vi "MeasureBreakdown.vi"(1 "Microsites":refnum<k24>, 2 "Junction Name":string, 7 ".NET Refnum":refnum<k24>, 9 "Function":string, 12 "appended path":path, 13 "new file path (Not A Path if cancelled)":path, 14 "UiDefinition":T1) -> (15 "error out":errorcluster)   [LabVIEW 2020]
uses:
  UIReferences.ctl
  D:/LabviewDXFViewer/LabviewDXFViewer/bin/Release/LabviewDXFViewer.exe
  LabviewDXFViewer/bin/Release/LabviewDXFViewer.exe
  <vilib>/Utility/file.llb/Write Delimited Spreadsheet (DBL).vi
  <vilib>/Utility/file.llb/Write Delimited Spreadsheet (string).vi
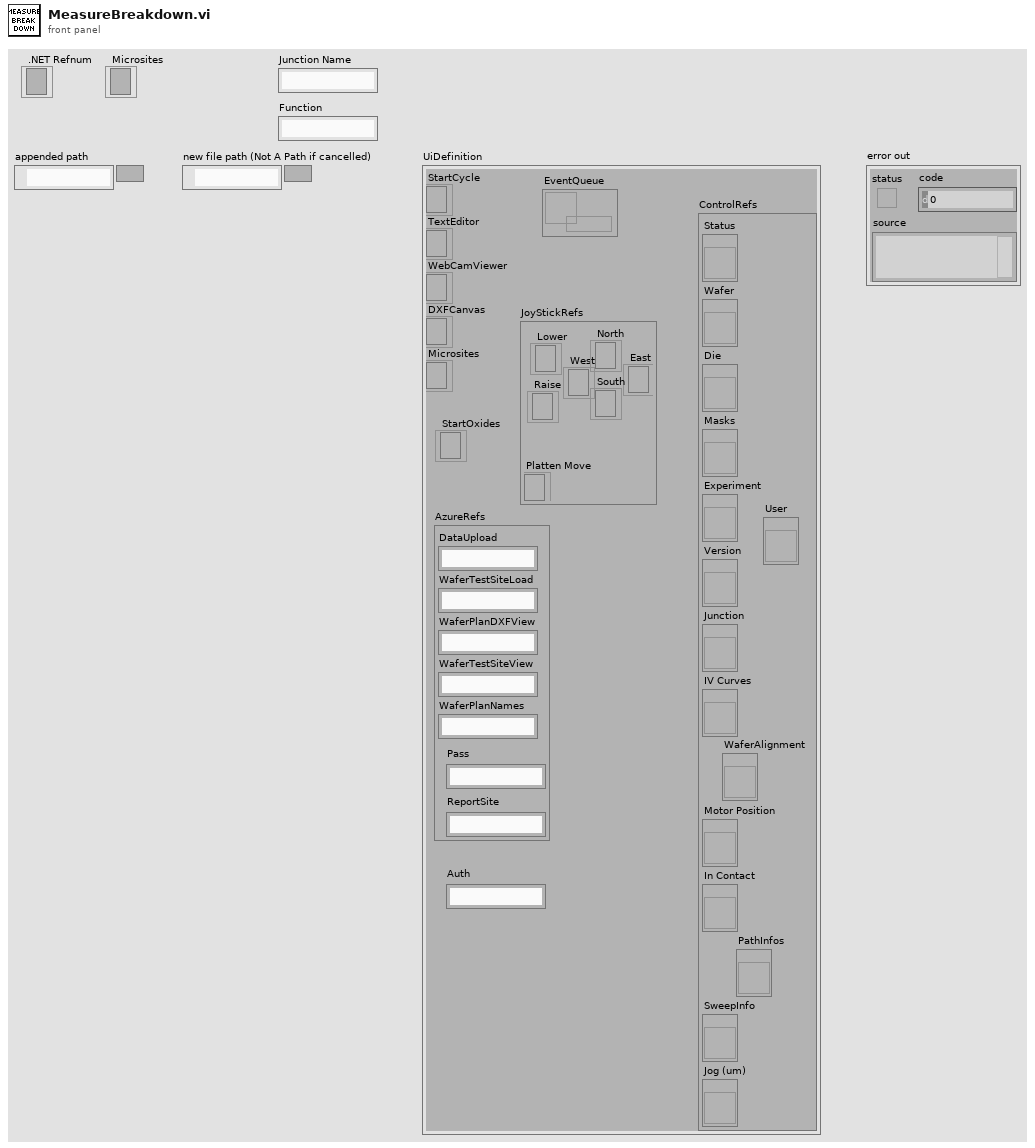
[diagram p1: front panel]
types:
  T1 = typedef "UIReferences.ctl" = cluster{"StartCycle":refnum<k24>, "TextEditor":refnum<k24>, "WebCamViewer":refnum<k24>, "DXFCanvas":refnum<k24>, "Microsites":refnum<k24>, "JoyStickRefs":cluster{"North":refnum<k24>, "Lower":refnum<k24>, "Raise":refnum<k24>, "Platten Move":refnum<k24>, "West":refnum<k24>, "East":refnum<k24>, "South":refnum<k24>}, "AzureRefs":cluster{"DataUpload":string, "WaferTestSiteLoad":string, "WaferPlanDXFView":string, "WaferTestSiteView":string, "WaferPlanNames":string, "Pass":string, "ReportSite":string}, "ControlRefs":cluster{"Status":refnum<vi>, "Wafer":refnum<vi>, "Die":refnum<vi>, "Masks":refnum<vi>, "Experiment":refnum<vi>, "Version":refnum<vi>, "Junction":refnum<vi>, "IV Curves":refnum<vi>, "Motor Position":refnum<vi>, "In Contact":refnum<vi>, "SweepInfo":refnum<vi>, "Jog (um)":refnum<vi>, "PathInfos":refnum<vi>, "User":refnum<vi>, "WaferAlignment":refnum<vi>}, "EventQueue":refnum<queue>, "StartOxides":refnum<k24>, "Auth":string}
  T2 = typedef "CapacitanceInfos.ctl" = cluster{"Conductance":dbl, "CapacitanceIV":dbl, "Intercept":dbl, "CapacitanceSW":dbl, "Sum":dbl, "CapacitanceInfos":T3[], "CapacitancePhase":dbl, "dC/dV":dbl, "Function":string, "OtherInfo":dbl[][]}
  T3 = typedef "CapacitanceRecord.ctl" = cluster{"Freq":dbl, "Vpp":dbl, "PhaseS":dbl, "Irms":dbl, "PhaseC":dbl, "Theta":dbl, "VDrive":dbl, "Capacitance":dbl, "Other":dbl}
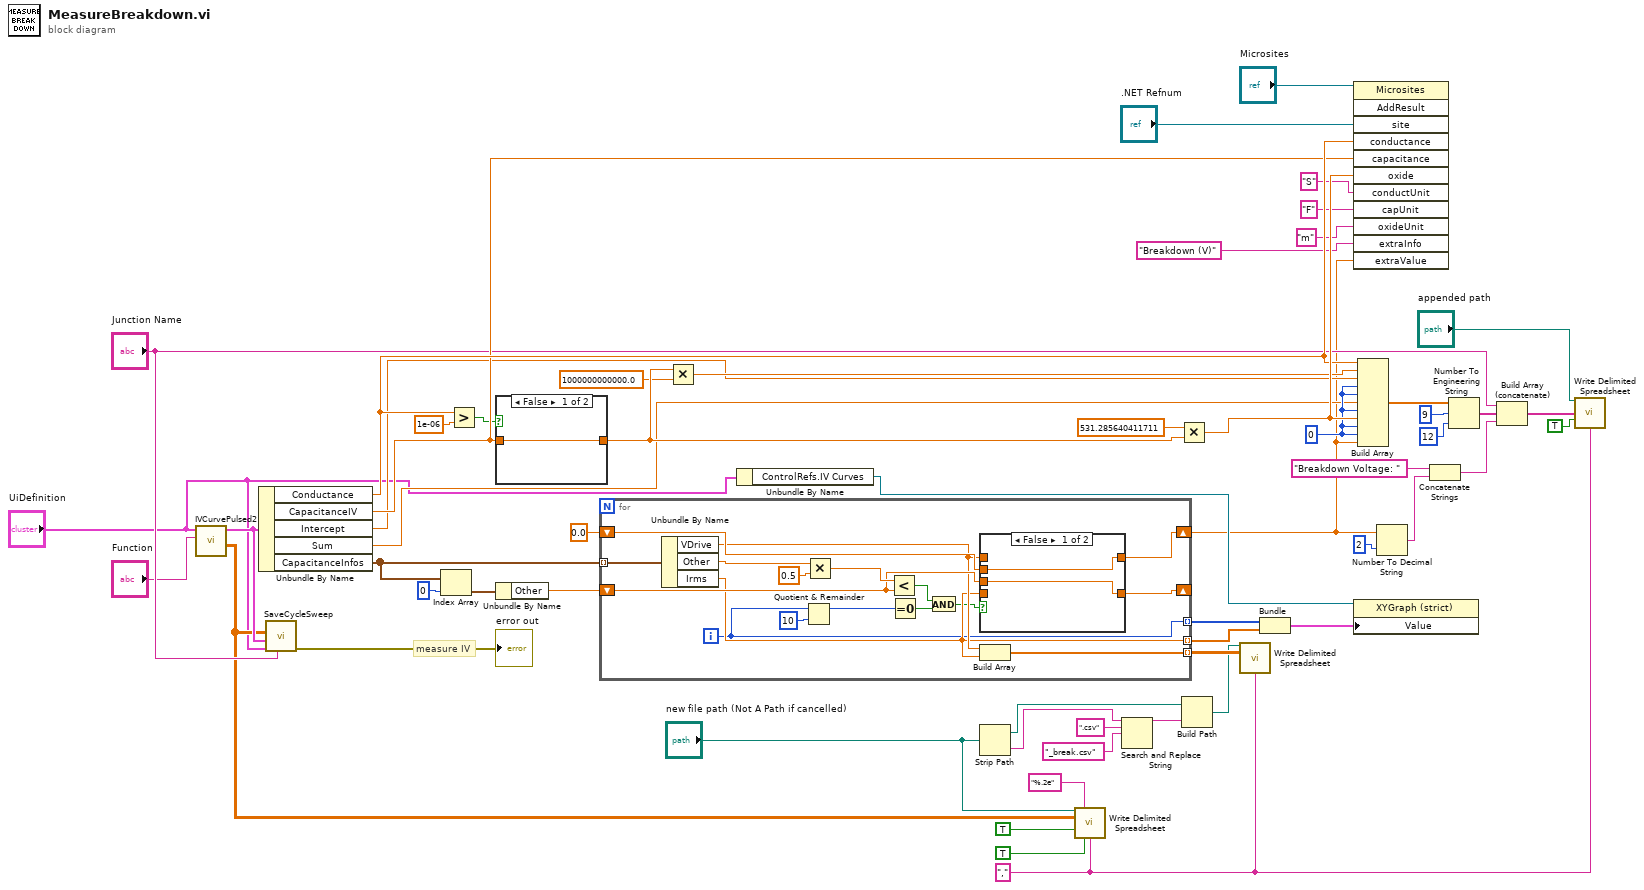
[diagram p0: block diagram]
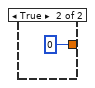
[diagram p3: hidden frame]
diagram:
  w17 = "," ("delimiter (\\t)")
  w47 = 0
  # "measure IV"
  n1 = call "IVCurvePulsed2.vi"("Program"="Function", "UiDefinition"="UiDefinition") -> ("appended array"=w26:dbl[][], "InfoCluster"=w39:T2)  [unwired: 8 in]
  n2 = Unbundle By Name(w39) -> ("Conductance"=w46:dbl, "CapacitanceIV"=w45:dbl, "Intercept"=w29:dbl, "Sum"=w30:dbl, "CapacitanceInfos"=w50:T3[])
  n3 = call "SaveCycleSweep.vi"("JunctionName"="Junction Name", "UiDefinition 2"="UiDefinition", "InfoCluster"=w39, "appended array"=w26) -> ("error out"=→"error out":errorcluster)  [unwired: 7 in]
  n4 = Index Array(array=w50, index=0) -> (element=w52:T3)
  n5 = Greater?(x=w46, y=1e-06) -> (0:w33:bool)
  n6 = case shown="False" w33 {
    tunnel: [w58 0] -> w56
    tunnel: w45 -> [w58 _]
    frame False {
    }
    frame True {
    }
  }
  n7 = Unbundle By Name(w52) -> ("Other"=w53:dbl)
  n8 = for {
    tunnel: w50 -> [w76] mode=indexing
    tunnel: [w64] -> w48 mode=indexing
    tunnel: [w65] -> w49 mode=indexing
    shift-right: [w69] -> _
    shift-left: w53 -> [w70]
    shift-right: [w74] -> w2
    shift-left: 0.0 ("Vpp") -> [w73]
    tunnel: [w66] -> w19 mode=indexing
    i -> [w64]
    n9 = Unbundle By Name(w76) -> ("VDrive"=w67:dbl, "Other"=w68:dbl, "Irms"=w65:dbl)
    n10 = Quotient & Remainder(x=w64, y=10) -> (x-y*floor(x/y)=w60:i32)  [unwired: 1 out]
    n11 = Multiply(x=w68, y=0.5) -> (x*y=w72:dbl)
    n12 = Less?(x=w72, y=w70) -> (x < y?=w75:bool)
    n13 = Equal To 0?(x=w60) -> (x = 0?=w61:bool)
    n14 = And(x=w75, y=w61) -> (x .and. y?=w62:bool)
    n15 = case shown="False" w62 {
      tunnel: w67 -> [_ w80]
      tunnel: [w78 w80] -> w74
      tunnel: w73 -> [w78 _]
      tunnel: [w77 w79] -> w69
      tunnel: w70 -> [w77 _]
      tunnel: w65 -> [_ w79]
      frame False {
      }
      frame True {
      }
    }
    n16 = Build Array(w67, w65) -> (w66:dbl[])
  }
  n17 = Multiply(x=w56, y=1000000000000.0) -> (x*y=w31:dbl)
  n18 = Unbundle By Name("UiDefinition") -> ("ControlRefs.IV Curves"=w8:refnum<vi>)
  n19 = Strip Path(path="new file path (Not A Path if cancelled)") -> (stripped path=w11:path, name=w15:string)
  n20 = call-poly <vilib>:"Write Delimited Spreadsheet.vi"("file path (dialog if empty)"="new file path (Not A Path if cancelled)", "format (%.3f)"="%.2e", "2D data"=w26, "append to file? (new file:F)"=TRUE, "transpose? (no:F)"=TRUE, "delimiter (\\t)"=w17) -> ()  [unwired: 8 in, 2 out]
  n21 = Search and Replace String(input string=w15, search string=".csv", replace string="_break.csv" ("replace string (\"\")")) -> (result string=w12:string)  [unwired: 5 in, 3 out]
  n22 = Multiply(x=531.285640411711, y=w56) -> (x*y=w57:dbl)
  n23 = Build Path(base path=w11, name or relative path=w12) -> (appended path=w10:path)
  n24 = call-poly <vilib>:"Write Delimited Spreadsheet.vi"("file path (dialog if empty)"=w10, "2D data"=w19, "delimiter (\\t)"=w17) -> ()  [unwired: 11 in, 2 out]
  n25 = Bundle(w48, w49) -> (w7:cluster{i32[], dbl[]})  [unwired: 1 in]
  n26 = invoke class="Microsites" method="AddResult"(reference="Microsites", "site"=".NET Refnum", "conductance"=w46, "capacitance"=w45, "oxide"=w57, "conductUnit"="S", "capUnit"="F", "oxideUnit"="m" ("interceptUnit"), "extraInfo"="Breakdown (V)", "extraValue"=w2) -> ()  [unwired: 2 in, 12 out]
  n27 = property class="XYGraph (strict)"(reference=w8, "Value"=w7) -> ()  [unwired: 1 in, 2 out]
  n28 = Build Array(w46, w31, w29, w47, w47, w30, w47, w57, w47, w47, w2) -> (w28:dbl[])
  n29 = Number To Decimal String(number=w2, width (-)=i16 2) -> (decimal integer string=w6:string)
  n30 = Concatenate Strings("Breakdown Voltage: ", w6) -> (w3:string)
  n31 = Number To Engineering String(2:i16 12 ("precision (6)"), 3:i16 9 ("width (-)"), 4:w28) -> (0:w20:string[])  [unwired: 1 in]
  n32 = Build Array (concatenate)("Junction Name", w20, w3) -> (w22:string[])
  n33 = call-poly <vilib>:"Write Delimited Spreadsheet.vi"("file path (dialog if empty)"="appended path", "1D data"=w22, "append to file? (new file:F)"=TRUE, "delimiter (\\t)"=w17) -> ()  [unwired: 10 in, 2 out]
